vi "InbitWait.vi"(1 "timeout":dbl=5.0 format="%0.2f", 2 "Inbit line":tag="6509/port0/line0") -> (0 "Timed out":bool=TRUE)   [LabVIEW 2018]
uses:
  <vilib>/DAQmx/read.llb/DAQmx Read (Digital Bool 1Line 1Point).vi
  <vilib>/DAQmx/create/channels.llb/DAQmx Create Channel (DI-Digital Input).vi
  <vilib>/DAQmx/miscellaneous.llb/DAQmx Fill In Error Info.vi
  <resource>/objmgr/daqmx.rc
panel:
  out "Value (no timeout)":bool
  out "Initialize (ms)":u32=4
  out "Read (ms)":u32=5003
  out "Clear (ms)":u32
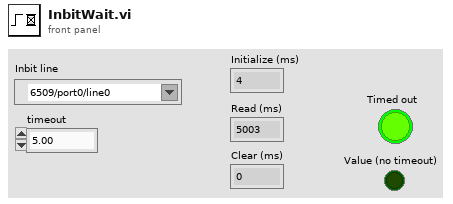
[diagram p1: front panel]
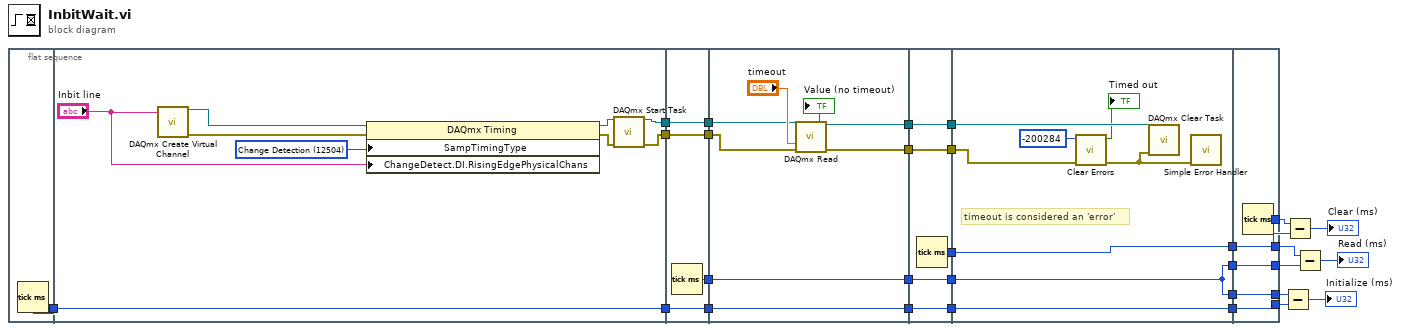
[diagram p0: block diagram]
diagram:
  n1 = flat-sequence {
    tunnel: [w30] -> w2
    tunnel: [w32] -> w29
    tunnel: [w35] -> w3
    tunnel: w2 -> [w35]
    tunnel: [w31] -> w1
    tunnel: w29 -> [w43]
    tunnel: [w43] -> w28
    tunnel: [w42] -> w27
    tunnel: [w41] -> w11
    tunnel: [w40] -> w4
    tunnel: w3 -> [w40]
    tunnel: w1 -> [w42]
    tunnel: w28 -> [w50]
    tunnel: w27 -> [w49]
    tunnel: [w48] -> w26
    tunnel: [w47] -> w24
    tunnel: [w46] -> w12
    tunnel: w11 -> [w46]
    tunnel: [w45] -> w5
    tunnel: w4 -> [w45]
    tunnel: w26 -> [w56]
    tunnel: [w56] -> w25
    tunnel: w24 -> [w55]
    tunnel: [w55] -> w23
    tunnel: [w54] -> w17
    tunnel: [w53] -> w13
    tunnel: w12 -> [w53]
    tunnel: [w52] -> w6
    tunnel: w5 -> [w52]
    tunnel: w25 -> [w61]
    tunnel: w23 -> [w63]
    tunnel: [w60] -> w18
    tunnel: w17 -> [w60]
    tunnel: [w59] -> w15
    tunnel: w13 -> [w59]
    tunnel: [w59] -> w10
    tunnel: [w58] -> w7
    tunnel: w6 -> [w58]
    tunnel: [w69] -> w19
    tunnel: [w68] -> w16
    tunnel: w18 -> [w68]
    tunnel: w15 -> [w67]
    tunnel: [w67] -> w14
    tunnel: w10 -> [w66]
    tunnel: [w66] -> w9
    tunnel: [w65] -> w8
    tunnel: w7 -> [w65]
    frame #0 {
      n2 = Tick Count (ms)() -> (millisecond timer value=w30:u32)
    }
    frame #1 {
      w37 = 12504 items=["Sample Clock"=10388, "Burst Handshake"=12548, "Handshake"=10389, "Implicit"=10451, "On Demand"=10390, "Change Detection"=12504, "Pipelined Sample Clock"=14668] ("SampTimingType")
      n3 = call-poly <vilib>:"DAQmx Create Virtual Channel.vi"("lines"="Inbit line") -> ("task out"=w38:refnum<k21>, "error out"=w39:errorcluster)  [unwired: 13 in]
      n4 = property class="DAQmx Timing"(reference=w38, error in=w39, "SampTimingType"=w37, "ChangeDetect.DI.RisingEdgePhysicalChans"="Inbit line") -> (reference out=w34:refnum<k21>, error out=w33:errorcluster)
      n5 = call <vilib>:"DAQmx Start Task.vi"("task/channels in"=w34, "error in"=w33) -> ("task out"=w32:refnum<k21>, "error out"=w31:errorcluster)  [unwired: 12 in]
    }
    frame #2 {
      n6 = Tick Count (ms)() -> (millisecond timer value=w41:u32)
    }
    frame #3 {
      n7 = call-poly <vilib>:"DAQmx Read.vi"("task/channels in"=w50, "timeout"="timeout", "error in"=w49) -> ("task out"=w48:refnum<k21>, "data"=→"Value (no timeout)":bool, "error out"=w47:errorcluster)  [unwired: 10 in]
    }
    frame #4 {
      n8 = Tick Count (ms)() -> (millisecond timer value=w54:u32)
    }
    frame #5 {
      # "timeout is considered an 'error'"
      n9 = call <vilib>:"Clear Errors.vi"("error in (no error)"=w63, "specific error code to clear (0: all)"=-200284) -> ("error out"=w64:errorcluster, "specific error cleared?"=→"Timed out":bool)  [unwired: 4 in]
      n10 = call <vilib>:"DAQmx Clear Task.vi"("task in"=w61, "error in"=w64) -> ()  [unwired: 13 in, 1 out]
      n11 = call <vilib>:"Simple Error Handler.vi"("error in (no error)"=w64) -> ()  [unwired: 4 in, 5 out]
    }
    frame #6 {
      n12 = Tick Count (ms)() -> (millisecond timer value=w69:u32)
    }
  }
  n13 = Subtract(x=w9, y=w8) -> (x-y=→"Initialize (ms)":u32)
  n14 = Subtract(x=w19, y=w16) -> (x-y=→"Clear (ms)":u32)
  n15 = Subtract(x=w16, y=w14) -> (x-y=→"Read (ms)":u32)
